vi "Config High Voltage.vi"(0 "VISA resource name":refnum<visa-resource-name>, 7 "High  Voltage Control (T:On)":bool=TRUE, 11 "error in (no error)":errorcluster) -> (4 "VISA resource name out":refnum<visa-resource-name>, 15 "error out":errorcluster)   [LabVIEW 2011, in "Stanford Research PS300 Series.lvlib"]
doc: "This VI controls the setting of high voltage switch on the front panel, turning the output voltage on or off.\n\nNotes*: If the front switch is in the OFF position, the high voltage is left off and an execution error is reported."
uses:
  <instrlib>/Stanford Research PS300 Series/Stanford Research PS300 Series.lvlib
panel:
  # "On\nOff"
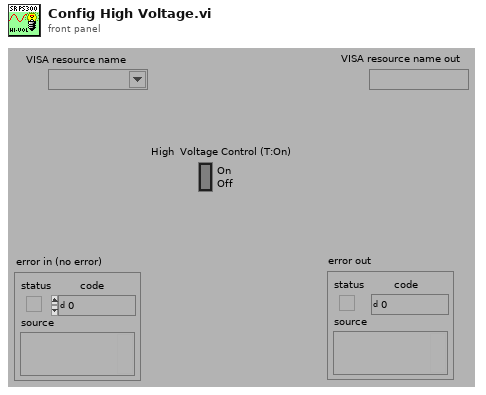
[diagram p1: front panel]
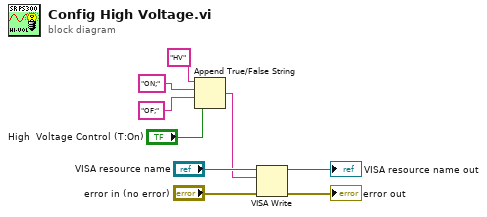
[diagram p0: block diagram]
diagram:
  n1 = Append True/False String(1:"High  Voltage Control (T:On)", 2:"OF;" ("false string"), 3:"ON;" ("true string"), 4:"HV" ("string (\"\")")) -> (0:w5:string)
  n2 = VISA Write(VISA resource name="VISA resource name", write buffer=w5, error in (no error)="error in (no error)") -> (VISA resource name out=→"VISA resource name out":refnum<visa-resource-name>, error out=→"error out":errorcluster)  [unwired: 1 out]
